vi "Connection.vi"(8 "error in (no error)":errorcluster, 11 "SerialResource in":refnum<class "SerialResource.lvclass">) -> (0 "error out":errorcluster, 2 "Connection":refnum<class "Connection.lvclass">, 3 "SerialResource out":refnum<class "SerialResource.lvclass">)   [LabVIEW 2020, in "PicoG-Core.lvlib" / "SerialResource.lvclass"]
uses:
  SerialResource.lvclass
  <vilib>/IlluminatedG/lv-stream/Connection/Connection.lvclass
  SerialResource.lvclass/SerialResource.ctl
  <vilib>/IlluminatedG/IG Serial Stream/Stream-Serial/Serial Client/Serial Client.lvclass
  C:/Program Files (x86)/National Instruments/LabVIEW 2020/vi.lib/IlluminatedG/lv-stream/Connection/Connection.lvclass
  C:/Program Files (x86)/National Instruments/LabVIEW 2020/vi.lib/IlluminatedG/lv-stream/Endpoint/Endpoint.lvclass
  C:/Program Files (x86)/National Instruments/LabVIEW 2020/vi.lib/IlluminatedG/IG Serial Stream/Stream-Serial/Serial Client/Serial Client.lvclass
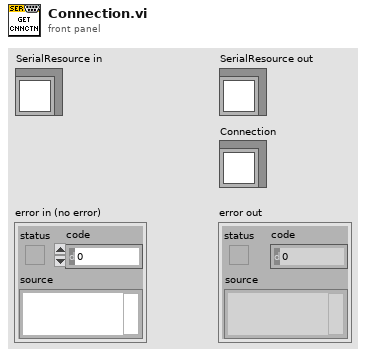
[diagram p1: front panel]
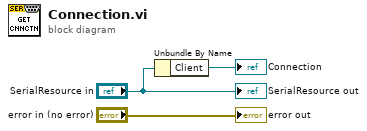
[diagram p0: block diagram]
diagram:
  n1 = Unbundle By Name("SerialResource in") -> ("Client"=→"Connection":refnum<class "Serial Client.lvclass">)
  "error out" <- "error in (no error)"
  "SerialResource out" <- "SerialResource in"
